vi "ReadElement.vi"(8 "error in (no error)":errorcluster, 10 "buffer location":u32, 11 "name":string) -> (0 "error out":errorcluster, 2 "found":bool, 3 "DVR element":T1)   [LabVIEW 2017, in "DVRBuffer.lvlib"]
uses:
  <vilib>/addons/InsightCM/Devices/Shared/Common/DVRBuffer/DVRBuffer.lvlib
  <vilib>/addons/InsightCM/Devices/Shared/Common/DVRBuffer/controls/DVRElement.ctl
  <vilib>/addons/InsightCM/Devices/Shared/Common/DVRBuffer/controls/DVRBuffer.ctl
  <vilib>/addons/PointValueMap/subVIs/Point_Read_variant.vi
  <vilib>/addons/PointValueMap/PointValueMap.lvlib
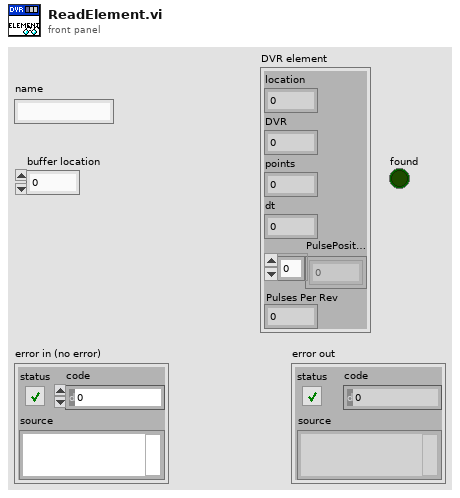
[diagram p1: front panel]
types:
  T1 = typedef "DVRBuffer.lvlib/DVRElement.ctl" = cluster{"location":u32, "DVR":u32, "points":i32, "dt":dbl, "PulsePositions":dbl[], "Pulses Per Rev":dbl}
  T2 = typedef "PointValueMap.lvlib/PointMap.ctl" = refnum<data-value>
  T3 = typedef "DVRBuffer.lvlib/DVRBuffer.ctl" = cluster{"buffer":T1[], "write ptr index":i32, "last block":u32, "buffer size":u32}
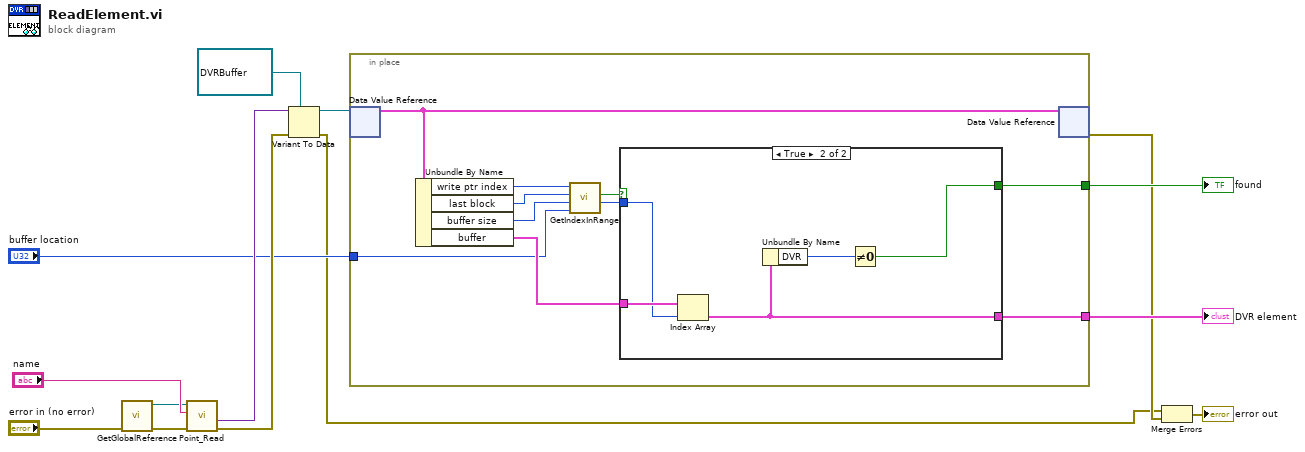
[diagram p0: block diagram]
diagram:
  n1 = call <vilib>:"GetGlobalReference.vi"("error in (no error)"="error in (no error)") -> ("error out"=w10:errorcluster, "reference"=w8:T2)  [unwired: 9 in]
  n2 = call-poly <vilib>:"Point_Read.vi"("Error In"=w10, "Tag"="name", "Map"=w8) -> ("Error Out"=w13:errorcluster, "Value"=w12:variant)  [unwired: 3 in, 4 out]
  n3 = Variant To Data(error in=w13, type=refnum<data-value> refnum ("data value reference"), Variant=w12) -> (data=w6:refnum<data-value>, error out=w1:errorcluster)
  n4 = in-place {
    in-place-border: "buffer location" -> [w16]
    in-place-border: [w22] -> w4
    in-place-border: [w21] -> w5
    n5 = in-place-dvr #1(w6) -> (w24:T3)  [unwired: 1 out]
    n6 = Unbundle By Name(w24) -> ("write ptr index"=w20:i32, "last block"=w19:u32, "buffer size"=w18:u32, "buffer"=w23:T1[])
    n7 = call <vilib>:"GetIndexInRange.vi"("location"=w16, "buffer size"=w18, "last block"=w19, "write pointer"=w20) -> ("index"=w15:i32, "in range"=w17:bool)  [unwired: 6 in]
    n8 = case shown="True" w17 {
      tunnel: w23 -> [_ w29]
      tunnel: [_ w27] -> w22
      tunnel: [_ w25] -> w21
      tunnel: w15 -> [_ w28]
      frame False {
      }
      frame True {
        n9 = Index Array(array=w29, index=w28) -> (element=w27:T1)
        n10 = Unbundle By Name(w27) -> ("DVR"=w26:u32)
        n11 = Not Equal To 0?(x=w26) -> (x != 0?=w25:bool)
      }
    }
    n12 = in-place-dvr #1(w24) -> (w3:errorcluster)  [unwired: 1 out]
  }
  "found" <- w5
  "DVR element" <- w4
  n13 = Merge Errors(w1, w3) -> (→"error out":errorcluster)
